vi "connect.vi"(8 "error in (no error)":errorcluster, 11 "SpectrographClientCommunicator in":refnum<class "SpectrographClientCommunicator.lvclass">) -> (0 "error out":errorcluster, 3 "SpectrographClientCommunicator out":refnum<class "SpectrographClientCommunicator.lvclass">)   [LabVIEW 2016, in "SpectrographClientCommunicator.lvclass"]
uses:
  SpectrographClientCommunicator.lvclass
  ts_labview_tcp/TCPClient/TCPClient.lvclass
panel:
  out "String":string
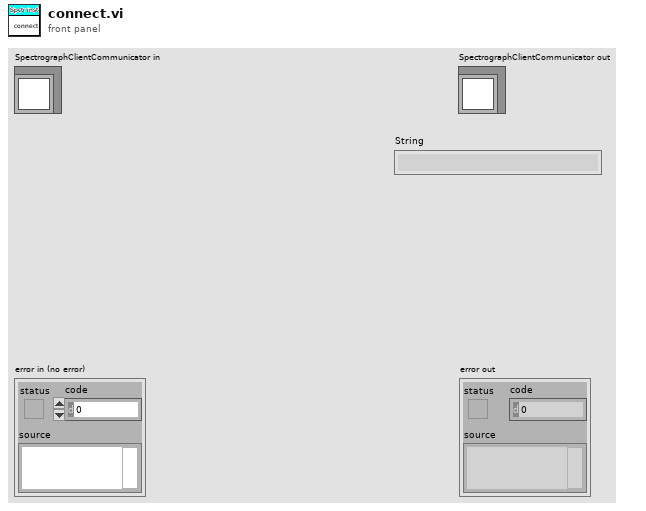
[diagram p1: front panel]
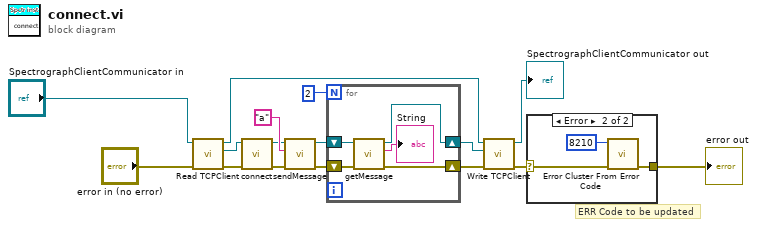
[diagram p0: block diagram]
diagram:
  # "ERR Code to be updated"
  n1 = call-dynamic "Read TCPClient.vi"("error in (no error)"="error in (no error)", "SpectrographClientCommunicator in"="SpectrographClientCommunicator in") -> ("error out"=w15:errorcluster, "TCPClient"=w16:refnum<class "TCPClient.lvclass">, "SpectrographClientCommunicator out"=w9:refnum<class "SpectrographClientCommunicator.lvclass">)  [unwired: 7 in]
  n2 = call-dynamic "connect.vi"("error in (no error)"=w15, "TCPClient in"=w16) -> ("error out"=w12:errorcluster, "TCPClient out"=w10:refnum<class "TCPClient.lvclass">)  [unwired: 8 in]
  n3 = call-dynamic "sendMessage.vi"("error in (no error)"=w12, "String"="a", "TCPClient in"=w10) -> ("error out"=w4:errorcluster, "TCPClient out"=w5:refnum<class "TCPClient.lvclass">)  [unwired: 7 in]
  n4 = for {
    N: 2 -> [_]
    shift-right: [w19] -> w3
    shift-left: w5 -> [w21]
    shift-right: [w18] -> w2
    shift-left: w4 -> [w20]
    n5 = call-dynamic "getMessage.vi"("error in (no error)"=w20, "TCPClient in"=w21) -> ("error out"=w18:errorcluster, "String"=→"String":string, "TCPClient out"=w19:refnum<class "TCPClient.lvclass">)  [unwired: 7 in]
  }
  n6 = call-dynamic "Write TCPClient.vi"("error in (no error)"=w2, "TCPClient"=w3, "SpectrographClientCommunicator in"=w9) -> ("error out"=w8:errorcluster, "SpectrographClientCommunicator out"=→"SpectrographClientCommunicator out":refnum<class "SpectrographClientCommunicator.lvclass">)  [unwired: 7 in]
  n7 = case shown="Error" w8 {
    selector: w8 -> [w22 w25]
    tunnel: [w22 w24] -> w6
    frame No Error {
    }
    frame Error {
      n8 = call <vilib>:"Error Cluster From Error Code.vi"("error in (no error)"=w25, "error code (0)"=8210) -> ("error out"=w24:errorcluster)  [unwired: 7 in]
    }
  }
  "error out" <- w6
